vi "Configure PA MESSAGE query.vi"(8 "error in (no error)":errorcluster, 10 "Step":T1=1 min=1 max=99 step=1, 11 "VISA resource in":refnum<visa-resource-name>) -> (0 "error out":errorcluster, 2 "Message":string, 3 "VISA resource out":refnum<visa-resource-name>)   [LabVIEW 2025, in "Chroma 19052.lvlib"]
uses:
  <instrlib>/Chroma 19052/Chroma 19052.lvlib
  <instrlib>/Chroma 19052/Public/Utility/Type Def/steps--numeric.ctl
  <vilib>/Utility/error.llb/Trim Whitespace One-Sided.vi
panel:
  # "Get PA Message query"
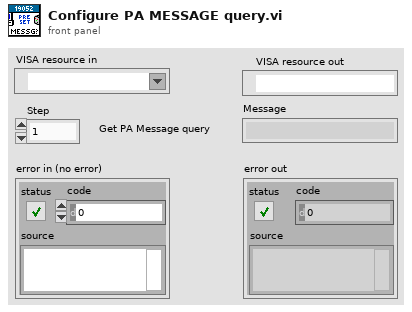
[diagram p1: front panel]
types:
  T1 = typedef "Chroma 19052.lvlib/steps--numeric.ctl" = u8
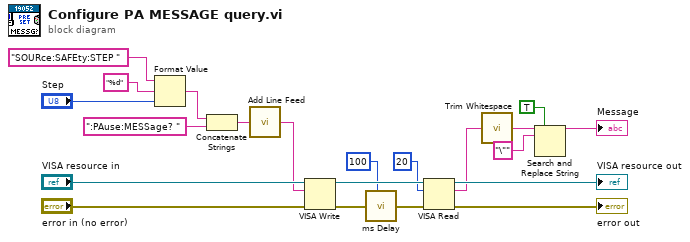
[diagram p0: block diagram]
diagram:
  n1 = Format Value(string ("")="SOURce:SAFEty:STEP ", format string="%d", value (0)="Step") -> (output string=w14:string)
  n2 = Concatenate Strings(w14, ":PAuse:MESSage? ") -> (w8:string)
  n3 = call <instrlib>:"Add Line Feed.vi"("Command string"=w8) -> ("Concatenated string"=w7:string)  [unwired: 4 in]
  n4 = VISA Write(VISA resource name="VISA resource in", write buffer=w7, error in (no error)="error in (no error)") -> (VISA resource name out=w13:refnum<visa-resource-name>, error out=w11:errorcluster)  [unwired: 1 out]
  n5 = call <instrlib>:"ms Delay.vi"("miliseconds to wait"=u32 100, "error in (no error)"=w11) -> ("error out"=w10:errorcluster)  [unwired: 6 in, 1 out]
  n6 = VISA Read(VISA resource name=w13, byte count=u32 20, error in (no error)=w10) -> (VISA resource name out=→"VISA resource out":refnum<visa-resource-name>, read buffer=w3:string, error out=→"error out":errorcluster)  [unwired: 1 out]
  n7 = call <vilib>:"Trim Whitespace.vi"("string"=w3) -> ("trimmed string"=w4:string)  [unwired: 1 in]
  n8 = Search and Replace String(replace all?=TRUE ("replace all? (F)"), input string=w4, search string="\"") -> (result string=→"Message":string)  [unwired: 5 in, 3 out]
